vi "CommonVIs_GetDatatypeFromString.vi"(0 "String":string, 7 "Classes":T1[](array[typedef]), 11 "error in (no error)":errorcluster) -> (4 "AttributeDataType":T2, 6 "ClassPath":path, 8 "ArrayDimensions":i32, 10 "DataTypeAsString(Array,default values removed)":string, 15 "error out":errorcluster)   [LabVIEW 2020]
uses:
  <resource>/Framework/Providers/Open_GDS/ClassProviders/Common/CommonVIs/CommonVIs_AttributeDataType.ctl
  <resource>/Framework/Providers/Open_GDS/ClassProviders/Common/CommonVIs/CommonVIs_ClassNamePathType.ctl
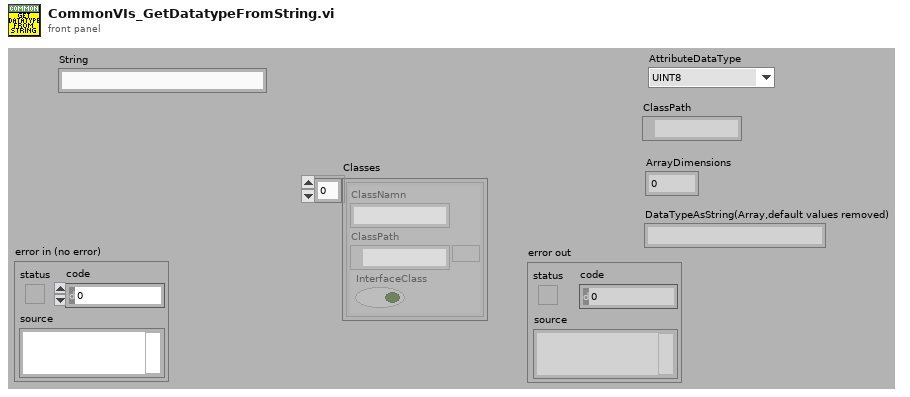
[diagram p1: front panel]
types:
  T1 = typedef "CommonVIs_ClassNamePathType.ctl" = cluster{"ClassNamn":string, "ClassPath":path, "InterfaceClass":bool}
  T2 = typedef "CommonVIs_AttributeDataType.ctl" = enum16{"UINT8", "INT8", "UINT16", "INT16", "UINT32", "INT32", "UINT64", "INT64", "SGL", "DBL", "EXT", "CSG", "CDB", "CXT", "TimeStamp", "STRING", "PATH", "BOOL", "ENUM", "RefNum", "VIRefNum", "LabVIEW Class", "Cluster", "Variant", "TypeDef", "Waveform", "LabVIEW Object", "Other", "void", "Set", "Map"}
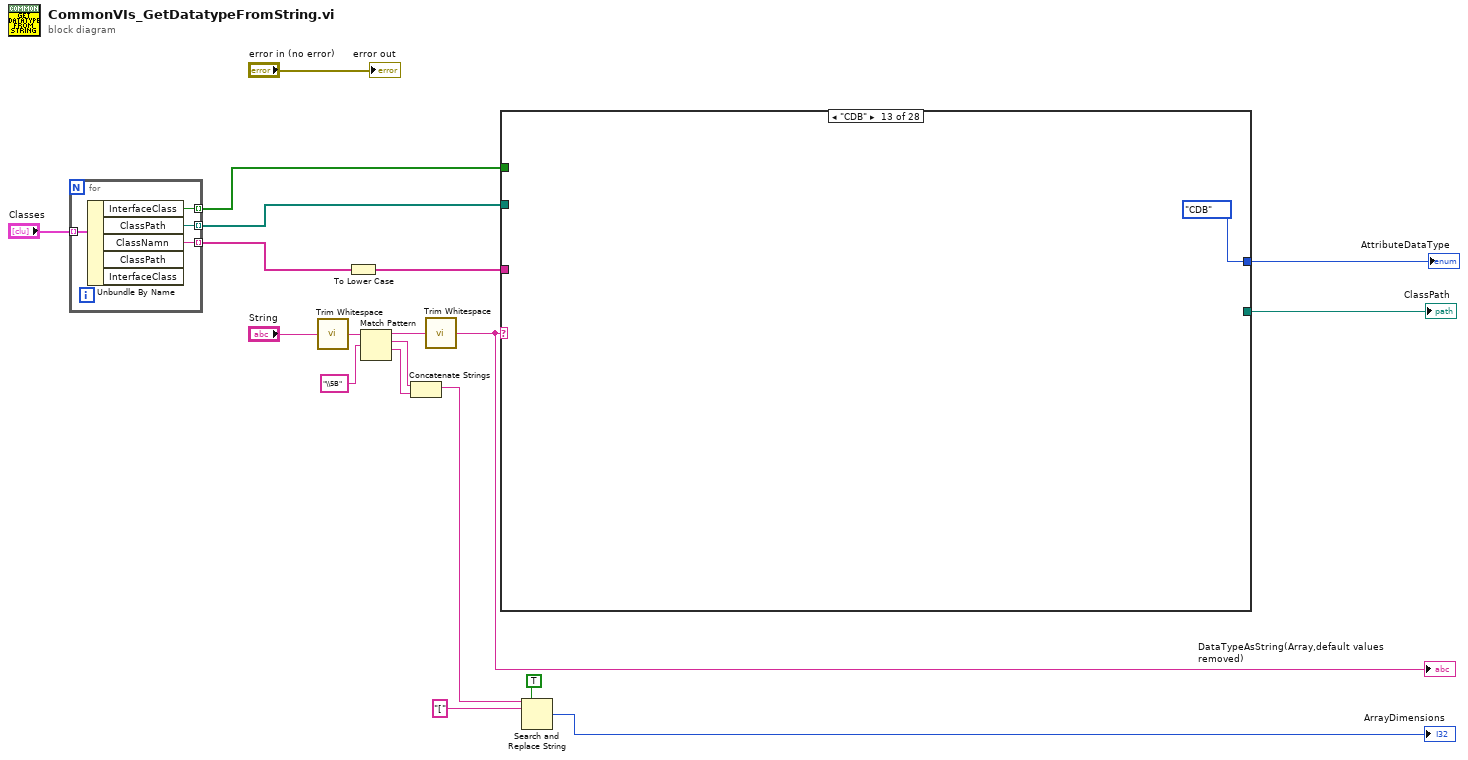
[diagram p0: block diagram]
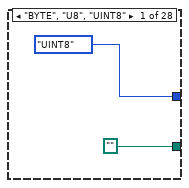
[diagram p2: hidden frame]
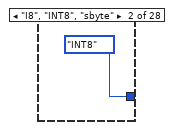
[diagram p3: hidden frame]
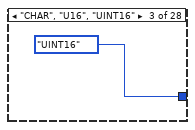
[diagram p4: hidden frame]
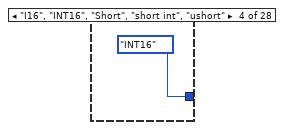
[diagram p5: hidden frame]
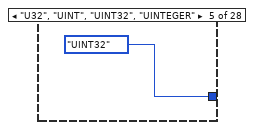
[diagram p6: hidden frame]
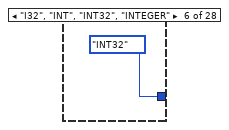
[diagram p7: hidden frame]
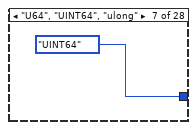
[diagram p8: hidden frame]
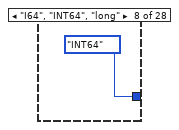
[diagram p9: hidden frame]
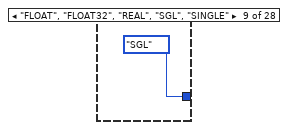
[diagram p10: hidden frame]
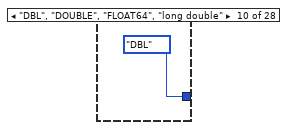
[diagram p11: hidden frame]
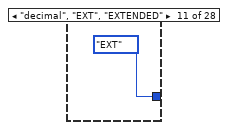
[diagram p12: hidden frame]
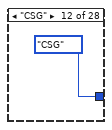
[diagram p13: hidden frame]
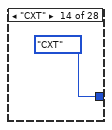
[diagram p14: hidden frame]
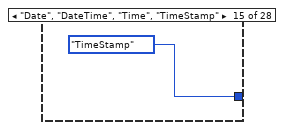
[diagram p15: hidden frame]
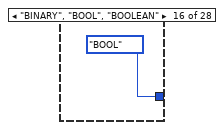
[diagram p16: hidden frame]
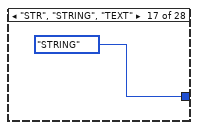
[diagram p17: hidden frame]
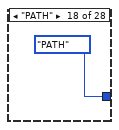
[diagram p18: hidden frame]
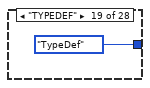
[diagram p19: hidden frame]
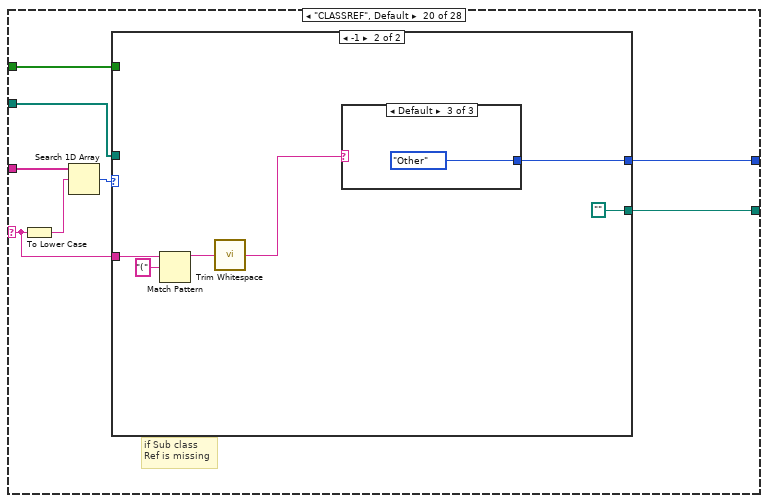
[diagram p20: hidden frame]
diagram:
  n1 = for {
    tunnel: "Classes" -> [w23] mode=indexing
    tunnel: [w22] -> w3 mode=indexing
    tunnel: [w21] -> w2 mode=indexing
    tunnel: [w20] -> w1 mode=indexing
    n2 = Unbundle By Name(w23) -> ("InterfaceClass"=w20:bool, "ClassPath"=w22:path, "ClassNamn"=w21:string)  [unwired: 2 out]
  }
  n3 = call <vilib>:"Trim Whitespace.vi"("string"="String") -> ("trimmed string"=w14:string)  [unwired: 1 in]
  n4 = To Lower Case(string=w2) -> (all lower case string=w11:string[])
  n5 = Match Pattern(string=w14, regular expression="\\5B") -> (before substring=w18:string, match substring=w10:string, after substring=w9:string)  [unwired: 2 out]
  n6 = Concatenate Strings(w10, w9) -> (w8:string)
  n7 = call <vilib>:"Trim Whitespace.vi"("string"=w18) -> ("trimmed string"=w19:string)  [unwired: 1 in]
  "DataTypeAsString(Array,default values removed)" <- w19
  n8 = case shown="\"CDB\"" w19 {
    selector: w19 -> [_ _ _ _ _ _ _ _ _ _ _ _ _ _ _ _ _ _ _ w44 _ _ _ _ _ _ _ _]
    tunnel: [CommonVIs_AttributeDataType."UINT8" ("AttributeDataType") CommonVIs_AttributeDataType."INT8" ("AttributeDataType") CommonVIs_AttributeDataType."UINT16" ("AttributeDataType") CommonVIs_AttributeDataType."INT16" ("AttributeDataType") CommonVIs_AttributeDataType."UINT32" ("AttributeDataType") CommonVIs_AttributeDataType."INT32" ("AttributeDataType") CommonVIs_AttributeDataType."UINT64" ("AttributeDataType") CommonVIs_AttributeDataType."INT64" ("AttributeDataType") CommonVIs_AttributeDataType."SGL" ("AttributeDataType") CommonVIs_AttributeDataType."DBL" ("AttributeDataType") CommonVIs_AttributeDataType."EXT" ("AttributeDataType") CommonVIs_AttributeDataType."CSG" ("AttributeDataType") CommonVIs_AttributeDataType."CDB" ("AttributeDataType") CommonVIs_AttributeDataType."CXT" ("AttributeDataType") CommonVIs_AttributeDataType."TimeStamp" ("AttributeDataType") CommonVIs_AttributeDataType."BOOL" ("AttributeDataType") CommonVIs_AttributeDataType."STRING" ("AttributeDataType") CommonVIs_AttributeDataType."PATH" ("AttributeDataType") CommonVIs_AttributeDataType."TypeDef" ("AttributeDataType") w51 CommonVIs_AttributeDataType."RefNum" ("AttributeDataType") CommonVIs_AttributeDataType."VIRefNum" ("AttributeDataType") CommonVIs_AttributeDataType."Variant" ("AttributeDataType") CommonVIs_AttributeDataType."ENUM" ("AttributeDataType") CommonVIs_AttributeDataType."Cluster" ("AttributeDataType") CommonVIs_AttributeDataType."Waveform" ("AttributeDataType") CommonVIs_AttributeDataType."LabVIEW Object" ("AttributeDataType") CommonVIs_AttributeDataType."void" ("AttributeDataType")] -> w15
    tunnel: [path "" _ _ _ _ _ _ _ _ _ _ _ _ _ _ _ _ _ _ w47 _ _ _ _ _ _ _ _] -> w16
    tunnel: w11 -> [_ _ _ _ _ _ _ _ _ _ _ _ _ _ _ _ _ _ _ w49 _ _ _ _ _ _ _ _]
    tunnel: w3 -> [_ _ _ _ _ _ _ _ _ _ _ _ _ _ _ _ _ _ _ w46 _ _ _ _ _ _ _ _]
    tunnel: w1 -> [_ _ _ _ _ _ _ _ _ _ _ _ _ _ _ _ _ _ _ w45 _ _ _ _ _ _ _ _]
    frame "BYTE", "U8", "UINT8" {
    }
    frame "I8", "INT8", "sbyte" {
    }
    frame "CHAR", "U16", "UINT16" {
    }
    frame "I16", "INT16", "Short", "short int", "ushort" {
    }
    frame "U32", "UINT", "UINT32", "UINTEGER" {
    }
    frame "I32", "INT", "INT32", "INTEGER" {
    }
    frame "U64", "UINT64", "ulong" {
    }
    frame "I64", "INT64", "long" {
    }
    frame "FLOAT", "FLOAT32", "REAL", "SGL", "SINGLE" {
    }
    frame "DBL", "DOUBLE", "FLOAT64", "long double" {
    }
    frame "decimal", "EXT", "EXTENDED" {
    }
    frame "CSG" {
    }
    frame "CDB" {
    }
    frame "CXT" {
    }
    frame "Date", "DateTime", "Time", "TimeStamp" {
    }
    frame "BINARY", "BOOL", "BOOLEAN" {
    }
    frame "STR", "STRING", "TEXT" {
    }
    frame "PATH" {
    }
    frame "TYPEDEF" {
    }
    frame "CLASSREF", Default {
      # "if Sub class\nRef is missing"
      n9 = To Lower Case(string=w44) -> (all lower case string=w50:string)
      n10 = Search 1D Array(1D array=w49, element=w50) -> (index of element=w48:i32)  [unwired: 1 out]
      n11 = case shown="-1" w48 {
        selector: w48 -> [w53 _]
        tunnel: [w57 w81] -> w51
        tunnel: [w55 path ""] -> w47
        tunnel: w46 -> [w58 _]
        tunnel: w45 -> [w54 _]
        tunnel: w44 -> [_ w80]
        frame 0, Default {
          n12 = Index Array(array=w58, index=w53) -> (element=w56:path)
          n13 = Index Array(array=w54, index=w53) -> (element=w52:bool)
          n14 = case shown="False" w52 {
            tunnel: [w61 CommonVIs_AttributeDataType."LabVIEW Object" ("DataType")] -> w57
            tunnel: w56 -> [w59 _]
            tunnel: [w60 _] -> w55
            frame False {
              n15 = Strip Path(path=w59) -> (name=w65:string)  [unwired: 1 out]
              n16 = Match Pattern(string=w65, regular expression="\\2E[Cc][Tt][Ll]$") -> (offset past match=w63:i32)  [unwired: 4 out]
              n17 = Greater Or Equal To 0?(x=w63) -> (x >= 0?=w62:bool)
              n18 = case shown="True" w62 {
                tunnel: [CommonVIs_AttributeDataType."LabVIEW Class" ("DataType") w72] -> w61
                tunnel: w59 -> [w68 w70]
                tunnel: [w67 w69] -> w60
                frame False {
                  n19 = call <resource>:"ReversedEngineering GetClassObjectRefPath.vi"("llbClassPath"=w68) -> ("classObjectRefPath"=w67:path)  [unwired: 1 in, 17 out]
                }
                frame True {
                  n20 = File/Directory Info(path=w70) -> (error out=w71:errorcluster)  [unwired: 1 in, 6 out]
                  n21 = case shown="No Error" w71 {
                    tunnel: [CommonVIs_AttributeDataType."TypeDef" ("DataType") CommonVIs_AttributeDataType."STRING" ("DataType")] -> w72
                    tunnel: w70 -> [w73 _]
                    tunnel: [w73 _] -> w69
                    frame No Error {
                    }
                    frame Error {
                    }
                  }
                }
              }
            }
            frame True {
            }
          }
        }
        frame -1 {
          n22 = Match Pattern(string=w80, regular expression="(") -> (before substring=w78:string)  [unwired: 4 out]
          n23 = call <vilib>:"Trim Whitespace.vi"("string"=w78) -> ("trimmed string"=w77:string)  [unwired: 1 in]
          n24 = case shown="Default" w77 {
            tunnel: [CommonVIs_AttributeDataType."Set" ("DataType") CommonVIs_AttributeDataType."Map" ("DataType") CommonVIs_AttributeDataType."Other" ("DataType")] -> w81
            frame "SET" {
            }
            frame "MAP" {
            }
            frame Default {
            }
          }
        }
      }
    }
    frame "REFNUM" {
      (unwired) CommonVIs_AttributeDataType."TypeDef" ("AttributeDataType")
    }
    frame "VI REF", "VI REFNUM", "VIREF", "VIREFNUM" {
    }
    frame "VARIANT" {
    }
    frame "ENUM" {
    }
    frame "CLUSTER" {
    }
    frame "Waveform" {
    }
    frame "class", "class object", "Labview", "LabVIEW Object", "LabVIEWObject", "lvclass", "object", "object ref" {
    }
    frame "void" {
    }
  }
  "ClassPath" <- w16
  "AttributeDataType" <- w15
  n25 = Search and Replace String(replace all?=TRUE ("replace all? (F)"), input string=w8, search string="[") -> (number of replacements=→"ArrayDimensions":i32)  [unwired: 5 in, 3 out]
  "error out" <- "error in (no error)"
